vi "CT-Create (Continuous).vi"(0 "HCT Runtime in":T1, 7 "F0 (Hz)":dbl, 9 "Fs (Hz)":dbl, 11 "error in (no error)":errorcluster) -> (4 "HCT Runtime out":T1, 8 "HCT":dbl[](array[numeric]), 15 "error out":errorcluster)   [LabVIEW 2015]
uses:
  CT-Runtime Data.ctl
  Utility VIs/Math VIs/Math-Uniform Random Number (I32, scalar).vi
  Utility VIs/Math VIs/LinSpace.vi
  Utility VIs/Math VIs/LinSpace (x0-dx-npts).vi
panel:
  in  "Npts":i32
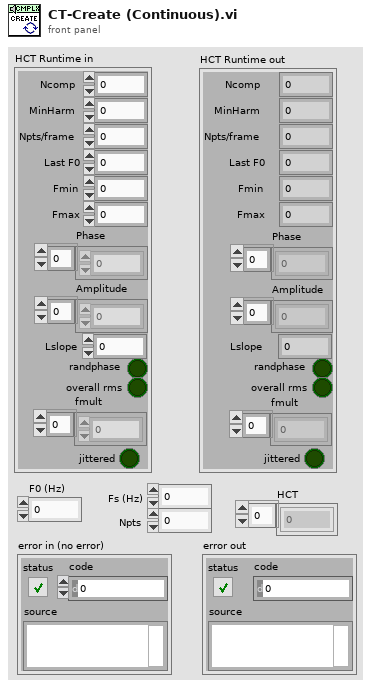
[diagram p1: front panel]
types:
  T1 = typedef "CT-Runtime Data.ctl" = cluster{"Ncomp":i32, "MinHarm":i32, "Phase":dbl[], "Amplitude":dbl[], "Npts/frame":i32, "Last F0":dbl, "Fmin":dbl, "Fmax":dbl, "Lslope":dbl, "randphase":bool, "overall rms":bool, "fmult":dbl[], "jittered":bool}
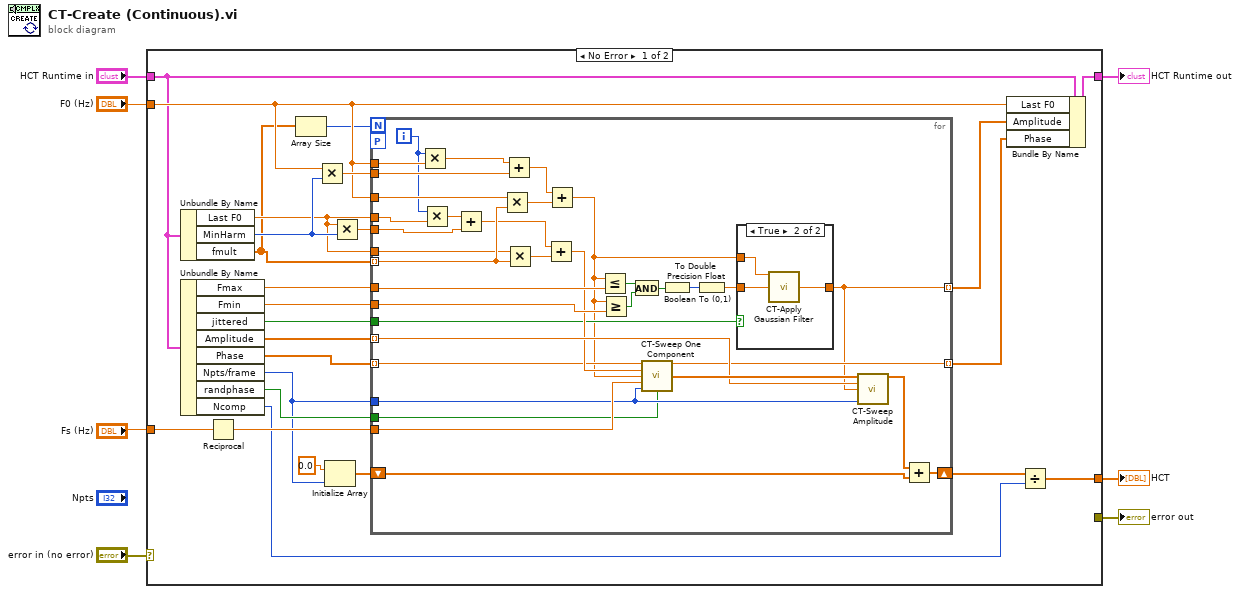
[diagram p0: block diagram]
diagram:
  n1 = case shown="No Error" "error in (no error)" {
    selector: "error in (no error)" -> [_ w72]
    tunnel: "HCT Runtime in" -> [w12 _]
    tunnel: [w27 _] -> w4
    tunnel: "F0 (Hz)" -> [w20 _]
    tunnel: [_ w72] -> w7
    tunnel: "Fs (Hz)" -> [w31 _]
    tunnel: [w24 _] -> w1
    frame No Error {
      n2 = Unbundle By Name(w12) -> ("Last F0"=w19:dbl, "MinHarm"=w23:i32, "fmult"=w14:dbl[])
      n3 = Unbundle By Name(w12) -> ("Fmax"=w29:dbl, "Fmin"=w28:dbl, "jittered"=w8:bool, "Amplitude"=w13:dbl[], "Phase"=w9:dbl[], "Npts/frame"=w18:i32, "randphase"=w21:bool, "Ncomp"=w22:i32)
      n4 = Reciprocal(x=w31) -> (1/x=w26:dbl)
      n5 = Array Size(array=w14) -> (size(s)=w17:i32)
      n6 = Multiply(x=w20, y=w23) -> (x*y=w32:dbl)
      n7 = Initialize Array(0.0 ("element"), w18) -> (w16:dbl[])
      n8 = Multiply(x=w19, y=w23) -> (x*y=w25:dbl)
      n9 = for {
        N: w17 -> [_]
        tunnel: w20 -> [w67]
        tunnel: w29 -> [w65]
        tunnel: w28 -> [w64]
        tunnel: w26 -> [w60]
        tunnel: w18 -> [w57]
        tunnel: w19 -> [w46]
        tunnel: w13 -> [w58] mode=indexing
        tunnel: w21 -> [w56]
        tunnel: w14 -> [w55] mode=indexing
        tunnel: w20 -> [w54]
        tunnel: w19 -> [w51]
        tunnel: w32 -> [w52]
        tunnel: w25 -> [w45]
        shift-right: [w42] -> w15
        shift-left: w16 -> [w40]
        tunnel: [w35] -> w11 mode=indexing
        tunnel: w9 -> [w38] mode=indexing
        tunnel: [w37] -> w10 mode=indexing
        workers-P: _ -> [_]
        tunnel: w8 -> [w36]
        i -> [w39]
        n10 = Multiply(x=w39, y=w67) -> (x*y=w48:dbl)
        n11 = Multiply(x=w39, y=w46) -> (x*y=w44:dbl)
        n12 = Add(x=w44, y=w45) -> (x+y=w43:dbl)
        n13 = Multiply(x=w54, y=w55) -> (x*y=w53:dbl)
        n14 = Add(x=w48, y=w52) -> (x+y=w47:dbl)
        n15 = Multiply(x=w51, y=w55) -> (x*y=w50:dbl)
        n16 = Add(x=w43, y=w50) -> (x+y=w49:dbl)
        n17 = Add(x=w47, y=w53) -> (x+y=w33:dbl)
        n18 = Less Or Equal?(x=w33, y=w65) -> (x <= y?=w63:bool)
        n19 = Greater Or Equal?(x=w33, y=w64) -> (x >= y?=w62:bool)
        n20 = And(x=w63, y=w62) -> (x .and. y?=w61:bool)
        n21 = call "CT-Sweep One Component.vi"("Phase In"=w38, "Last Freq (Hz)"=w49, "New Freq (Hz)"=w33, "dt (s)"=w60, "Npts"=w57, "randomize phase"=w56) -> ("Phase Out"=w37:dbl, "Y"=w59:dbl[])  [unwired: 8 in]
        n22 = Boolean To (0,1)(Boolean=w61) -> (0, 1=w66:i16)
        n23 = To Double Precision Float(number=w66) -> (double precision float=w34:dbl)
        n24 = case shown="True" w36 {
          tunnel: [w68 w69] -> w35
          tunnel: w34 -> [w68 w70]
          tunnel: w33 -> [_ w71]
          frame False {
          }
          frame True {
            n25 = call "CT-Apply Gaussian Filter.vi"("Freq (Hz)"=w71, "Amplitude in"=w70) -> ("Amplitude out"=w69:dbl)  [unwired: 13 in]
          }
        }
        n26 = call "CT-Sweep Amplitude.vi"("Y In"=w59, "Astart"=w58, "Aend"=w35, "Npts"=w57) -> ("Y Out"=w41:dbl[])  [unwired: 11 in]
        n27 = Add(x=w41, y=w40) -> (x+y=w42:dbl[])
      }
      n28 = Bundle By Name(cluster=w12, "Last F0"=w20, "Amplitude"=w11, "Phase"=w10) -> (w27:T1)
      n29 = Divide(x=w15, y=w22) -> (x/y=w24:dbl[])
    }
    frame Error {
    }
  }
  "error out" <- w7
  "HCT Runtime out" <- w4
  "HCT" <- w1
